vi "intento Señal cuadrada.vi"() -> ()   [LabVIEW 2023]
doc: "This example demonstrates how to generate a PWM signal on a single channel using a LINX device."
uses:
  <vilib>/MakerHub/LINX/Public/Peripherals/Digital/Digital Write 1 Chan.vi
  <vilib>/MakerHub/LINX/Public/Peripherals/Digital/Digital Write N Chans.vi
  <vilib>/MakerHub/LINX/Private/Local IO/LinxDigitalWrite.vi
  <vilib>/MakerHub/LINX/Public/Utilities/Check Channel.vi
  <vilib>/MakerHub/LINX/Public/Utilities/Open Serial.vi
  <vilib>/Waveform/DWDTOps.llb/DWDT Analog to Digital.vi
  <vilib>/Waveform/DWDTOps.llb/DWDT Digital to Boolean Array.vi
  <vilib>/MakerHub/LINX/Private/Utilties/Generate Error.vi
  <vilib>/MakerHub/LINX/LMH-LINX.lvlib
  <vilib>/Analysis/NI_AALBase.lvlib
panel:
  in  "amplitude":dbl=1.0 format="%0.2f"
  in  "delay":i32(slide) scale=0.0..2000.0
  in  "Canal de Control":u8=3
  in  "Stop Button":bool
  in  "Puerto Serie":refnum<visa-resource-name>
  # "Microcontrolador"
  # "Control mediante Señal Booleana para motor Paso a Paso\n\nEn este programa se controlara un programa para controlar un motor paso a paso mediante,\nuna señal cuadrada y convertida a valores booleanos.\nHay que tener en cuenta que cada valor logico equivale a un paso del motor, por lo que cuando\nponga un bit a uno y le de un tiempo para volver a cero , con ese flanco de subida indico un paso,\npor lo que a más frecuencia menor tiempo entre paso y paso, y por lo tanto mas velocidad.\n\nInstructions\n1. Seleccione El puerto Serie asociado con el microcontrolador.\n2. Seleccione El canal de control.\n3. Indique la Frecuencia para regular la velocidad."
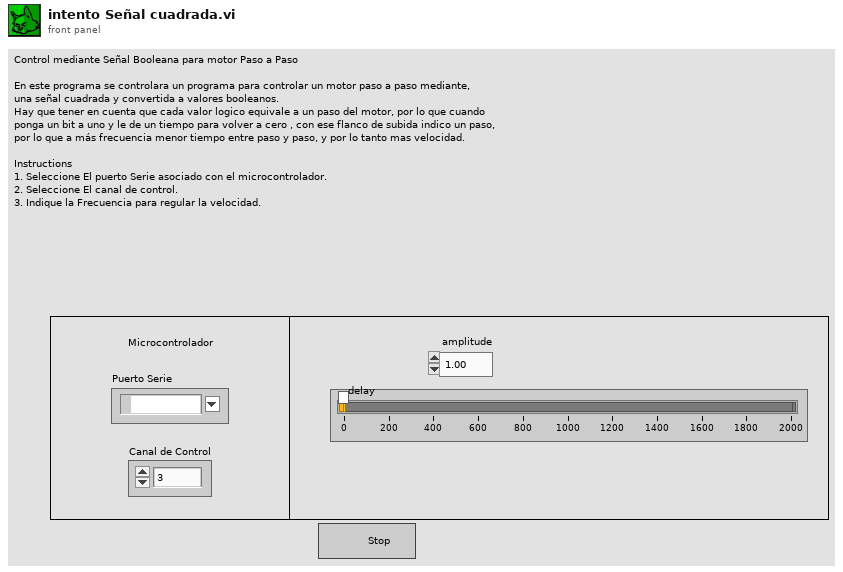
[diagram p1: front panel]
types:
  T1 = typedef "LMH-LINX.lvlib/LINX Ref.ctl" = cluster{"IO":T2, "Interface":T3, "LINX Device Config":T4}
  T2 = typedef "LMH-LINX.lvlib/Platform.ctl" = enum16{"Remote", "Local"}
  T3 = typedef "LMH-LINX.lvlib/Interface.ctl" = enum16{"Serial", "TCP"}
  T4 = typedef "LMH-LINX.lvlib/Device.lvlib/LINX Device Config.ctl" = cluster{"Interface":T3, "COM Port":refnum<visa-resource-name>, "TCP Configuration":T5, "Device Family":u8, "Device ID":u8, "Device Name":string, "TCP Ref":refnum<k5>, "Channels":T6}
  T5 = typedef "LMH-LINX.lvlib/Device.lvlib/TCP Config.ctl" = cluster{"IP Address":string, "Port":u16}
  T6 = typedef "LMH-LINX.lvlib/Channels.ctl" = cluster{"DI":u8[], "DO":u8[], "AI":u8[], "AO":u8[], "PWM":u8[], "QE":u8[], "UART":u8[], "I2C 2":u8[], "SPI":u8[], "CAN":u8[], "Servo":u8[], "AI Ref (V)":dbl, "AI Resolution (Bits)":u8, "AO Ref (V)":dbl, "AO Resolution (Bits)":u8}
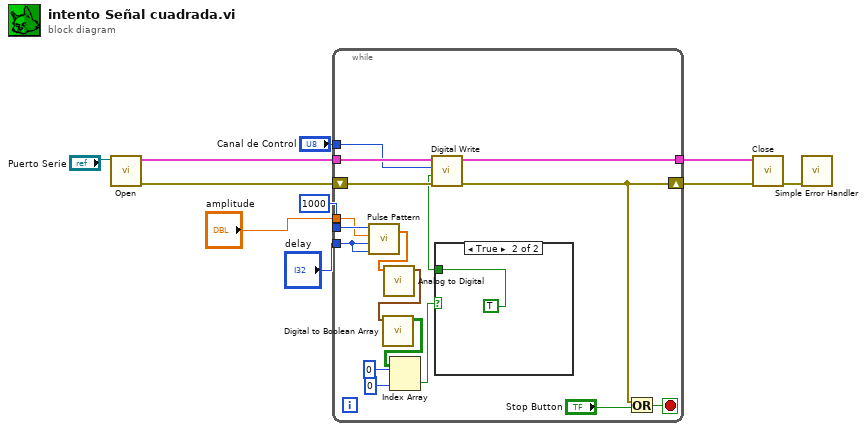
[diagram p0: block diagram]
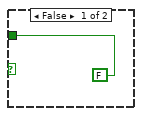
[diagram p2: hidden frame]
diagram:
  n1 = call-poly <vilib>:"Open.vi"("Serial Port"="Puerto Serie") -> ("Error Out"=w9:errorcluster, "LINX Resource"=w10:T1)  [unwired: 8 in, 1 out]
  n2 = while {
    tunnel: w10 -> [w24]
    shift-right: [w22] -> w8
    shift-left: w9 -> [w23]
    tunnel: "Canal de Control" -> [w21]
    tunnel: [w25] -> w4
    tunnel: "delay" -> [w11]
    tunnel: 1000 ("samples") -> [w13]
    tunnel: "amplitude" -> [w12]
    stop <- w27 stop-if-true
    n3 = call <vilib>:"Pulse Pattern.vi"("width"=w11, "delay"=w11, "amplitude"=w12, "samples"=w13) -> ("Pulse Pattern"=w14:dbl[])  [unwired: 1 out]
    n4 = call-poly <vilib>:"Analog to Digital.vi"("analog waveform"=w14) -> ("digital waveform"=w15:digitalwaveform)  [unwired: 7 in, 3 out]
    n5 = call-poly <vilib>:"Digital to Boolean Array.vi"("digital waveform"=w15) -> ("boolean array"=w17:bool[][])  [unwired: 9 in, 1 out]
    n6 = Index Array(array=w17, index (row)=0, index (col)=0 ("disabled index (col)")) -> (element=w16:bool)
    n7 = case shown="True" w16 {
      tunnel: [FALSE TRUE] -> w20
      frame False {
      }
      frame True {
      }
    }
    n8 = call-poly <vilib>:"Digital Write.vi"("Error In"=w23, "Output Value"=w20, "DO Channel"=w21, "LINX Resource"=w24) -> ("Error Out"=w22:errorcluster, "LINX Resource"=w25:T1)  [unwired: 6 in]
    n9 = Or(x=w22, y="Stop Button") -> (x .or. y?=w27:bool)
  }
  n10 = call <vilib>:"Close.vi"("Error In"=w8, "LINX Resource"=w4) -> ("Error Out"=w6:errorcluster)  [unwired: 9 in]
  n11 = call <vilib>:"Simple Error Handler.vi"("error in (no error)"=w6) -> ()  [unwired: 4 in, 5 out]
